vi "Queue_Initialization.vi"() -> ()   [LabVIEW 2024]
uses:
  typedeff_AnalisisQueue_cluster.ctl
  typedeff_DecisionQueue_cluster.ctl
panel:
  in  "DecisionQueue_cluster":T1
  in  "Analisis_Queue_cluster":T2
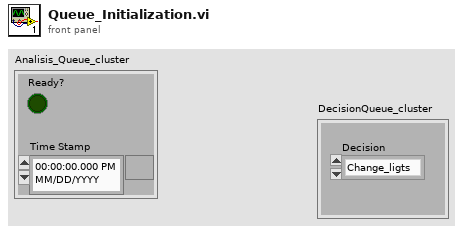
[diagram p1: front panel]
types:
  T1 = typedef "typedeff_DecisionQueue_cluster.ctl" = cluster{"Decision":enum16{"Change_ligts", "Wait"}}
  T2 = typedef "typedeff_AnalisisQueue_cluster.ctl" = cluster{"Ready?":bool, "Time Stamp":timestamp}
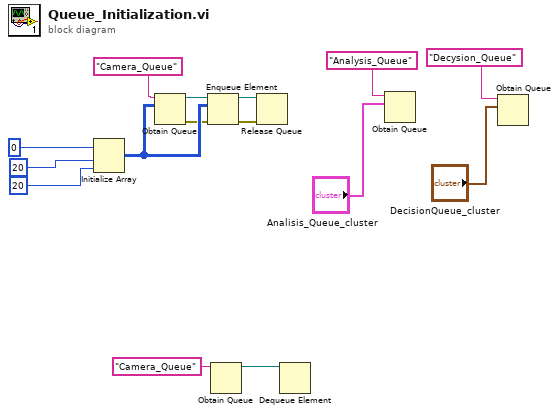
[diagram p0: block diagram]
diagram:
  n1 = Initialize Array(u8 0 ("element"), 20 ("dimension size"), 20 ("dimension size")) -> (w7:u8[][])
  n2 = Obtain Queue(name (unnamed)="Camera_Queue", element data type=w7) -> (queue out=w8:refnum<queue>, error out=w6:errorcluster)  [unwired: 3 in, 1 out]
  n3 = Enqueue Element(queue=w8, element=w7, error in (no error)=w6) -> (queue out=w4:refnum<queue>, error out=w3:errorcluster)  [unwired: 1 in, 1 out]
  n4 = Obtain Queue(name (unnamed)="Camera_Queue") -> (queue out=w1:refnum<queue>)  [unwired: 4 in, 2 out]
  n5 = Release Queue(queue=w4, error in (no error)=w3) -> ()  [unwired: 1 in, 3 out]
  n6 = Dequeue Element(queue=w1) -> ()  [unwired: 2 in, 4 out]
  n7 = Obtain Queue(name (unnamed)="Analysis_Queue", element data type="Analisis_Queue_cluster") -> ()  [unwired: 3 in, 3 out]
  n8 = Obtain Queue(name (unnamed)="Decysion_Queue", element data type="DecisionQueue_cluster") -> ()  [unwired: 3 in, 3 out]
